vi "Write clFlagImpairConfig.vi"(8 "error in (no error)":errorcluster, 10 "clFlagImpairConfig":T1, 11 "FlagImpairPluginBase in":refnum<class "FlagImpairPluginBase.lvclass">) -> (0 "error out":errorcluster, 3 "FlagImpairPluginBase out":refnum<class "FlagImpairPluginBase.lvclass">)   [LabVIEW 2017, in "FlagImpairPlugins.lvlib" / "FlagImpairPluginBase.lvclass"]
uses:
  FlagImpairPluginBase.lvclass
  TypeDefs/clFlagImpairConfig.ctl
  FlagImpairPluginBase.lvclass/FlagImpairPluginBase.ctl
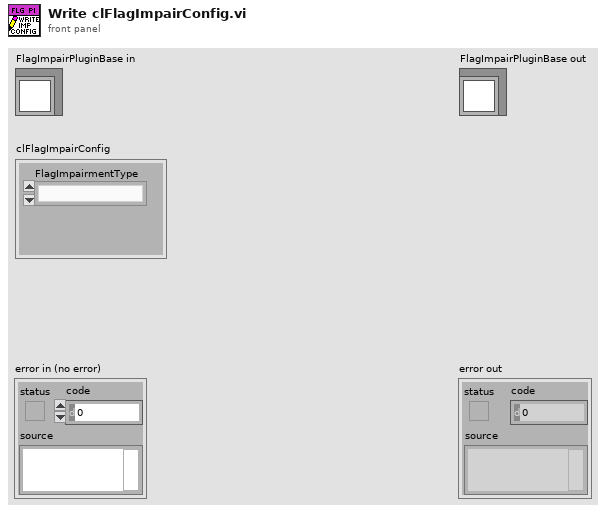
[diagram p1: front panel]
types:
  T1 = typedef "FlagImpairPlugins.lvlib/FlagImpairPluginBase.lvclass/clFlagImpairConfig.ctl" = cluster{"FlagImpairmentType":u16}
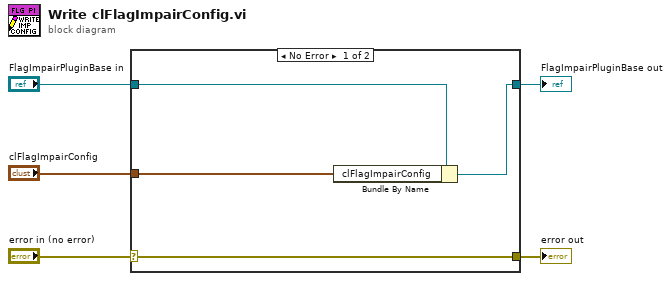
[diagram p0: block diagram]
diagram:
  n1 = case shown="No Error" "error in (no error)" {
    selector: "error in (no error)" -> [w9 w10]
    tunnel: [w9 w10] -> w4
    tunnel: [w7 w11] -> w2
    tunnel: "FlagImpairPluginBase in" -> [w8 w11]
    tunnel: "clFlagImpairConfig" -> [w6 _]
    frame No Error {
      n2 = Bundle By Name(cluster=w8, "clFlagImpairConfig"=w6) -> (w7:refnum<class "FlagImpairPluginBase.lvclass">)
    }
    frame Error {
    }
  }
  "error out" <- w4
  "FlagImpairPluginBase out" <- w2
